vi "Setup TestRunner Library.vi"(5 "Interactive (T)":bool=TRUE, 7 "Verbose (F)":bool, 8 "error in (no error)":errorcluster, 9 "Test Report":refnum<class "Test Report.lvclass">, 10 "Library Refnum":refnum<vi>, 11 "Test Runner.Library in":refnum<class "Test Runner.Library.lvclass">) -> (0 "error out":errorcluster, 3 "Test Runner.Library out":refnum<class "Test Runner.Library.lvclass">)   [LabVIEW 2020, in "Caraya.lvlib" / "Test Runner.Library.lvclass"]
uses:
  Test Runner.Library.lvclass
  C:/projects/caraya/src/classes/Test Runner/Test Runner.lvclass
  Test Report/Test Report.lvclass
  Test Runner/Test Runner.lvclass/Test Runner.ctl
  Test Runner.Library.lvclass/Test Runner.Library.ctl
  Test Runner/Test Runner.lvclass
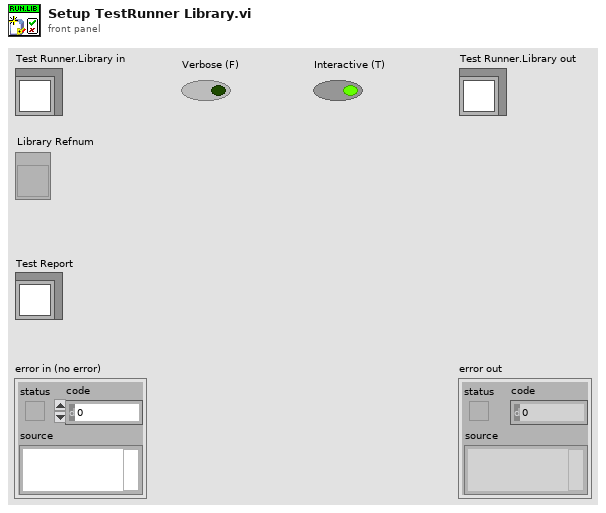
[diagram p1: front panel]
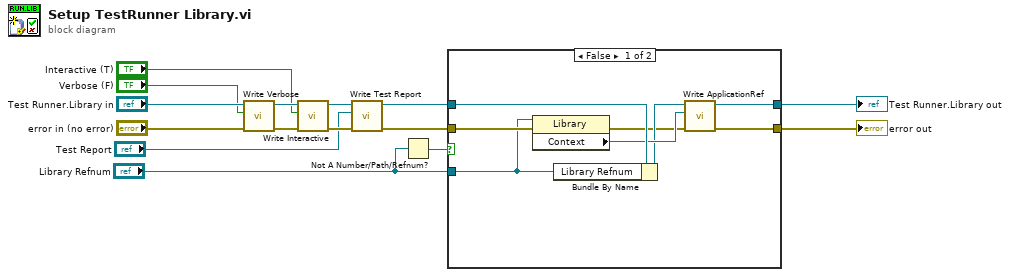
[diagram p0: block diagram]
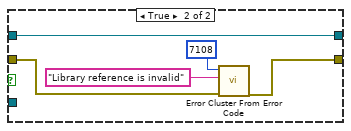
[diagram p2: hidden frame]
diagram:
  n1 = call "Write Verbose.vi"("Verbose"="Verbose (F)", "Test Runner in"="Test Runner.Library in") -> ("Test Runner out"=w10:refnum<class "Test Runner.Library.lvclass">)  [unwired: 9 in]
  n2 = call "Write Interactive.vi"("Interactive"="Interactive (T)", "Test Runner in"=w10) -> ("Test Runner out"=w9:refnum<class "Test Runner.Library.lvclass">)  [unwired: 9 in]
  n3 = call "Write Test Report.vi"("Test Report"="Test Report", "Test Runner in"=w9) -> ("Test Runner out"=w12:refnum<class "Test Runner.Library.lvclass">)  [unwired: 9 in]
  n4 = Not A Number/Path/Refnum?(number/path/refnum="Library Refnum") -> (NaN/Path/Refnum?=w11:bool)
  n5 = case shown="False" w11 {
    tunnel: w12 -> [w20 w21]
    tunnel: "error in (no error)" -> [w15 w23]
    tunnel: [w17 w21] -> w2
    tunnel: [w14 w22] -> w1
    tunnel: "Library Refnum" -> [w13 _]
    frame False {
      n6 = property class="Library"(reference=w13, error in=w15) -> (error out=w16:errorcluster, "Context"=w19:refnum<vi>)  [unwired: 1 out]
      n7 = Bundle By Name(cluster=w20, "Library Refnum"=w13) -> (w18:refnum<class "Test Runner.Library.lvclass">)
      n8 = call "Write ApplicationRef.vi"("error in (no error)"=w16, "Application"=w19, "Test Runner in"=w18) -> ("error out"=w14:errorcluster, "Test Runner out"=w17:refnum<class "Test Runner.Library.lvclass">)  [unwired: 7 in]
    }
    frame True {
      n9 = call <vilib>:"Error Cluster From Error Code.vi"("error in (no error)"=w23, "error message (\"\")"="Library reference is invalid" ("error message (\"\")"), "error code (0)"=7108) -> ("error out"=w22:errorcluster)  [unwired: 6 in]
    }
  }
  "error out" <- w1
  "Test Runner.Library out" <- w2
